vi "LAB1_SIGNAL_AND_SYSTEM.vi"() -> ()   [LabVIEW 2019]
uses:
  <vilib>/measure/maspectr.llb/FFT Spectrum (Mag-Phase) for 1 Chan.vi
  <vilib>/Analysis/NI_AALBase.lvlib
  <vilib>/measure/NI_MAPro.lvlib
  <vilib>/measure/NI_MABase.lvlib
panel:
  in  "stop":bool
  out "Frequancy domain":cluster{"f0":dbl, "df":dbl, "magnitude":dbl[]}(graph)
  in  "Function selection":T1(ring)
  in  "sampling information":cluster{"Fs":dbl, "#sample ":dbl}
  in  "Sine phase":dbl
  in  "Sine amplitude":dbl
  in  "Sine frequancy":dbl
  in  "Unit impulse and step delay":dbl
  out "Time domain":waveform(dbl)(graph)
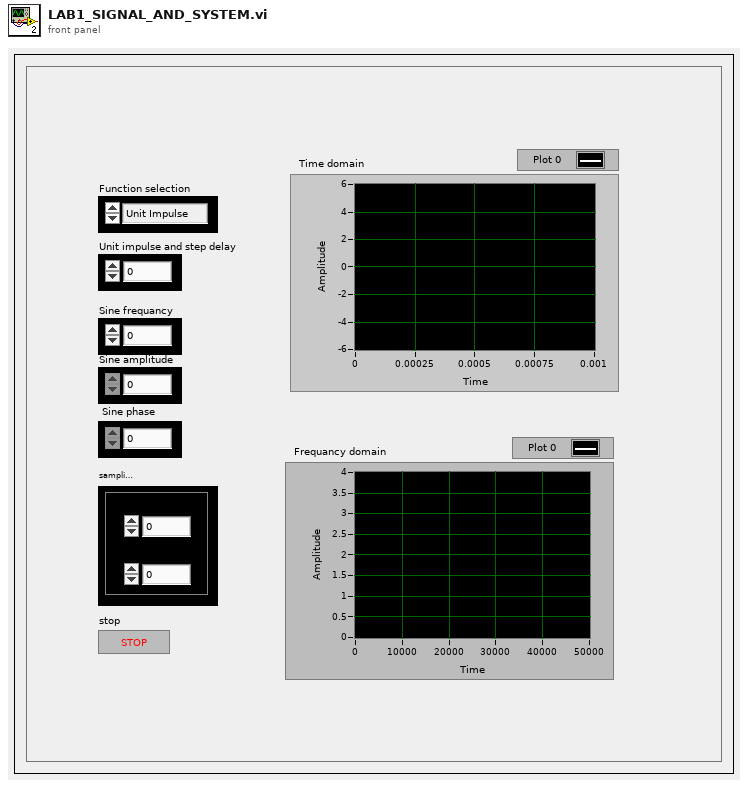
[diagram p1: front panel]
types:
  T1 = enum16{"Unit Impulse", "Unit step", "Sine", "AWGN"}
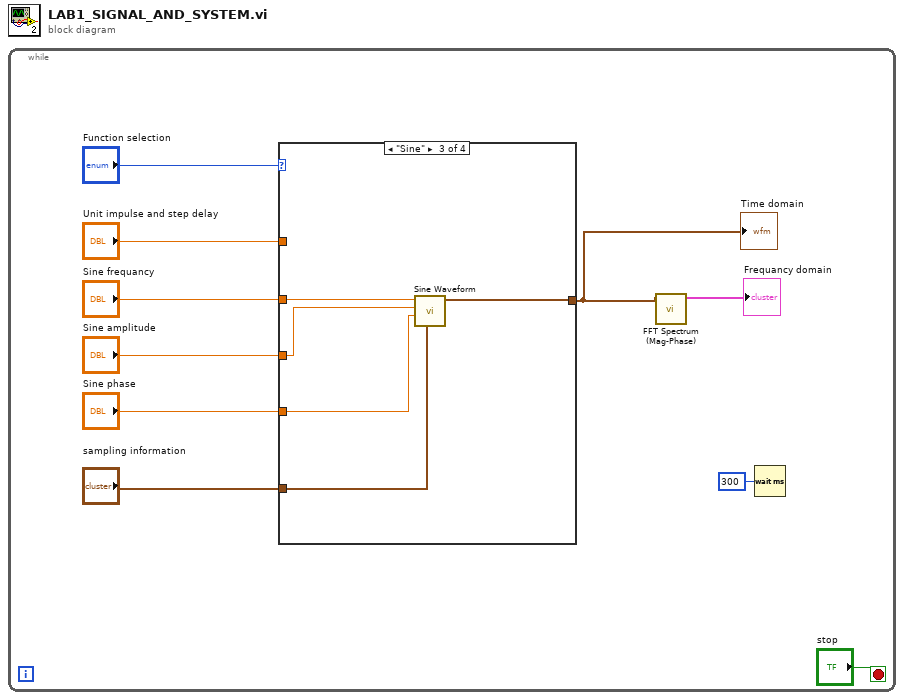
[diagram p0: block diagram]
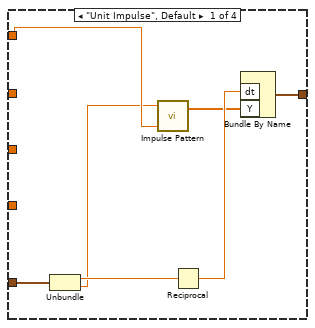
[diagram p2: hidden frame]
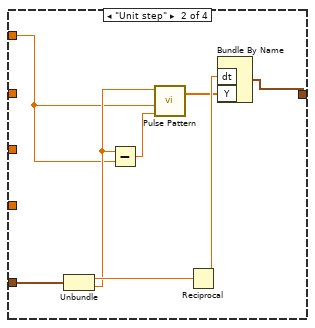
[diagram p3: hidden frame]
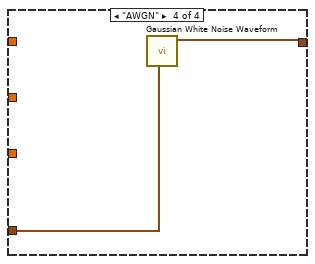
[diagram p4: hidden frame]
diagram:
  n1 = while {
    stop <- "stop" stop-if-true
    n2 = case shown="\"Sine\"" "Function selection" {
      tunnel: "sampling information" -> [w13 w22 w29 w32]
      tunnel: "Unit impulse and step delay" -> [w15 w19 _ _]
      tunnel: "Sine frequancy" -> [_ _ w30 _]
      tunnel: "Sine amplitude" -> [_ _ w28 _]
      tunnel: "Sine phase" -> [_ _ w27 _]
      tunnel: [w12 w18 w26 w31] -> w1
      frame "Unit Impulse", Default {
        n3 = Unbundle(w13) -> ("Fs"=w14:dbl, "#sample"=w11:dbl)
        n4 = call <vilib>:"Impulse Pattern.vi"("delay"=w15, "samples"=w11) -> ("Impulse Pattern"=w16:dbl[])  [unwired: 1 in, 1 out]
        n5 = Reciprocal(x=w14) -> (1/x=w17:dbl)
        n6 = Bundle By Name("dt"=w17, "Y"=w16) -> (w12:waveform(dbl))  [unwired: 1 in]
      }
      frame "Unit step" {
        n7 = Unbundle(w22) -> ("Fs"=w23:dbl, "#sample"=w20:dbl)
        n8 = Subtract(x=w20, y=w19) -> (x-y=w21:dbl)
        n9 = call <vilib>:"Pulse Pattern.vi"("width"=w21, "delay"=w19, "samples"=w20) -> ("Pulse Pattern"=w24:dbl[])  [unwired: 1 in, 1 out]
        n10 = Reciprocal(x=w23) -> (1/x=w25:dbl)
        n11 = Bundle By Name("dt"=w25, "Y"=w24) -> (w18:waveform(dbl))  [unwired: 1 in]
      }
      frame "Sine" {
        n12 = call <vilib>:"Sine Waveform.vi"("sampling info"=w29, "phase"=w27, "amplitude"=w28, "frequency"=w30) -> ("signal out"=w26:waveform(dbl))  [unwired: 6 in, 1 out]
      }
      frame "AWGN" {
        n13 = call <vilib>:"Gaussian White Noise Waveform.vi"("sampling info"=w32) -> ("signal out"=w31:waveform(dbl))  [unwired: 9 in, 1 out]
      }
    }
    "Time domain" <- w1
    n14 = call-poly <vilib>:"FFT Spectrum (Mag-Phase).vi"("time signal"=w1) -> ("magnitude"=→"Frequancy domain":cluster{"f0":dbl, "df":dbl, "magnitude":dbl[]})  [unwired: 6 in, 4 out]
    n15 = Wait (ms)(milliseconds to wait=u32 300) -> ()  [unwired: 1 out]
  }
